vi "Error Check Chassis Master.vi"(8 "error in (no error)":errorcluster, 10 "Connection Settings":T2, 11 "Item Ref in":T1 format="%.0x") -> (0 "error out":errorcluster, 3 "Item Ref out":T1 format="%.0x")   [LabVIEW 2020, in "NI Synchronization System Explorer.lvlib"]
uses:
  NI Synchronization System Explorer.lvlib
  Shared/Connection Settings.ctl
  Shared/Mode.ctl
  Shared/External Pin.ctl
  Shared/Routes.ctl
  Shared/Route.ctl
  <vilib>/NI VeriStand/Custom Device API/Custom Device Item Ref.ctl
  Shared/Constants.vi
  <vilib>/NI VeriStand/Custom Device API/Custom Device API.lvlib
  Shared/NI Synchronization Shared.lvlib
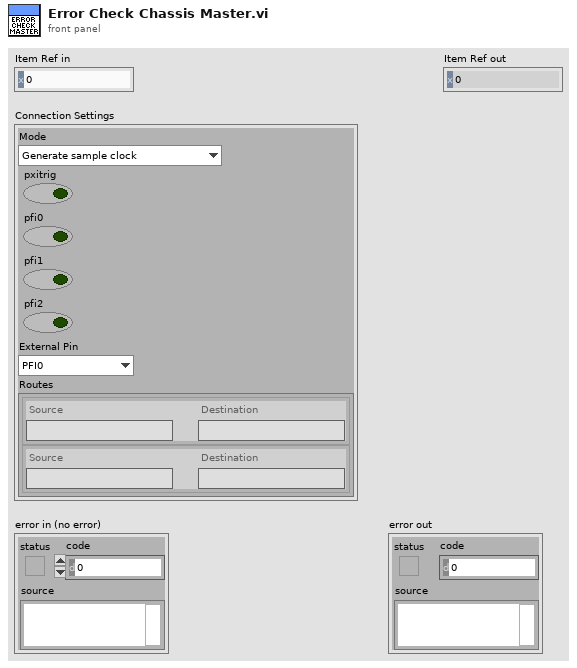
[diagram p1: front panel]
types:
  T1 = typedef "Custom Device API.lvlib/Custom Device Item Ref.ctl" = u64
  T2 = typedef "NI Synchronization Shared.lvlib/Connection Settings.ctl" = cluster{"Mode":T3, "pxitrig":bool, "pfi0":bool, "pfi1":bool, "pfi2":bool, "External Pin":T4, "Routes":T5}
  T3 = typedef "NI Synchronization Shared.lvlib/Mode.ctl" = enum16{"Generate sample clock", "Route sample clock out of chassis", "Route sample clock into chassis", "Custom routes"}
  T4 = typedef "NI Synchronization Shared.lvlib/External Pin.ctl" = enum16{"PFI0", "PFI1", "PFI2"}
  T5 = typedef "NI Synchronization Shared.lvlib/Routes.ctl" = T6[]
  T6 = typedef "NI Synchronization Shared.lvlib/Route.ctl" = cluster{"Source":string, "Destination":string}
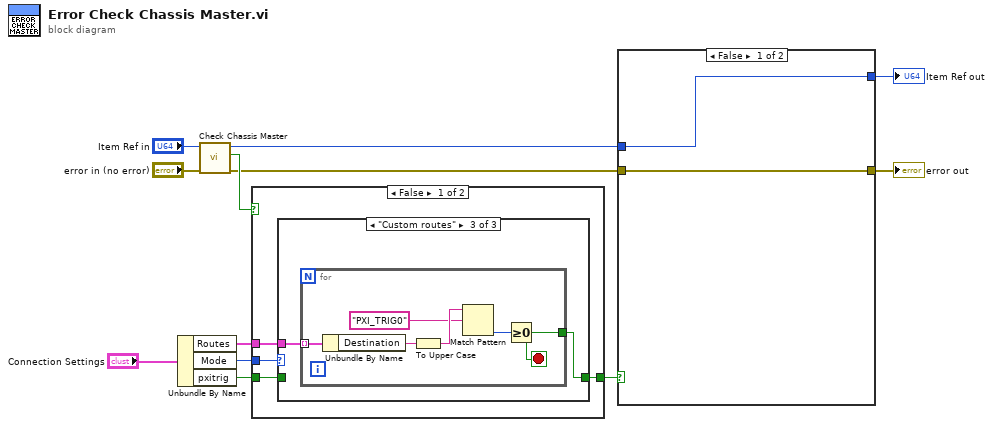
[diagram p0: block diagram]
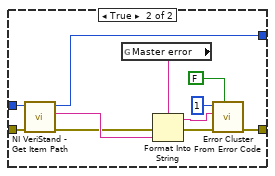
[diagram p2: hidden frame]
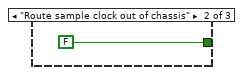
[diagram p4: hidden frame]
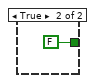
[diagram p5: hidden frame]
diagram:
  n1 = Unbundle By Name("Connection Settings") -> ("Routes"=w2:T5, "Mode"=w8:T3, "pxitrig"=w4:bool)
  n2 = call "Check Chassis Master.vi"("error in (no error)"="error in (no error)", "Device Item Ref in"="Item Ref in") -> ("error out"=w3:errorcluster, "Master?"=w9:bool, "Item Ref out"=w5:T1)  [unwired: 7 in]
  n3 = case shown="False" w9 {
    tunnel: w8 -> [w16 _]
    tunnel: [w15 FALSE] -> w6
    tunnel: w4 -> [w14 _]
    tunnel: w2 -> [w13 _]
    frame False {
      n4 = case shown="\"Custom routes\"" w16 {
        tunnel: [w17 FALSE ("pxitrig") w19] -> w15
        tunnel: w14 -> [w17 _ _]
        tunnel: w13 -> [_ _ w20]
        frame "Generate sample clock", "Route sample clock into chassis" {
        }
        frame "Route sample clock out of chassis" {
        }
        frame "Custom routes" {
          n5 = for {
            tunnel: w20 -> [w26] mode=indexing
            tunnel: [w21] -> w19
            stop <- w21 stop-if-true
            n6 = Unbundle By Name(w26) -> ("Destination"=w25:string)
            n7 = To Upper Case(1:w25) -> (0:w24:string)
            n8 = Match Pattern(string=w24, regular expression="PXI_TRIG0") -> (offset past match=w22:i32)  [unwired: 1 in, 3 out]
            n9 = Greater Or Equal To 0?(x=w22) -> (x >= 0?=w21:bool)
          }
        }
      }
    }
    frame True {
    }
  }
  n10 = case shown="False" w6 {
    tunnel: w3 -> [w29 w36]
    tunnel: [w29 w40] -> w7
    tunnel: w5 -> [w28 w35]
    tunnel: [w28 w30] -> w1
    frame False {
    }
    frame True {
      n11 = call <vilib>:"NI VeriStand - Get Item Path.vi"("error in (no error)"=w36, "Item Ref in"=w35) -> ("error out"=w33:errorcluster, "Path"=w34:string, "Item Ref out"=w30:T1)  [unwired: 6 in, 1 out]
      n12 = global read "Constants.vi" "Master error"() -> (w31:string)
      n13 = Format Into String(format string=w31, error in=w33, w34) -> (resulting string=w32:string, error out=w37:errorcluster)  [unwired: 1 in]
      n14 = call <vilib>:"Error Cluster From Error Code.vi"("show call chain? (False)"=FALSE, "error in (no error)"=w37, "error message (\"\")"=w32, "error code (0)"=1) -> ("error out"=w40:errorcluster)  [unwired: 5 in]
    }
  }
  "error out" <- w7
  "Item Ref out" <- w1
